vi "fgv_2470-config.vi"(7 "cmd":T2, 11 "2470-config":T1={"Source Mode"=enum."Voltage", "Source Limit Level"=0.01, "Source Level"=0.0, "Output_2470"=FALSE}) -> (3 "2470-config 2":T1)   [LabVIEW 2019]
uses:
  _ctrl/rw.ctl
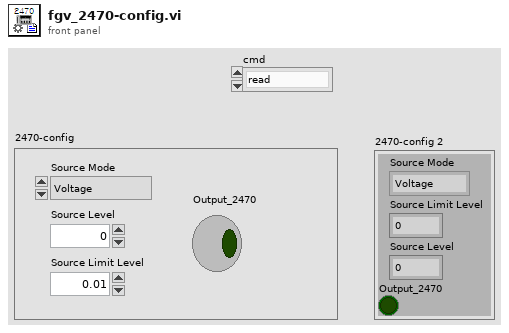
[diagram p1: front panel]
types:
  T1 = cluster{"Source Mode":enum16{"Voltage", "Current"}, "Source Limit Level":dbl, "Source Level":dbl, "Output_2470":bool}
  T2 = typedef "rw.ctl" = enum16{"read", "write"}
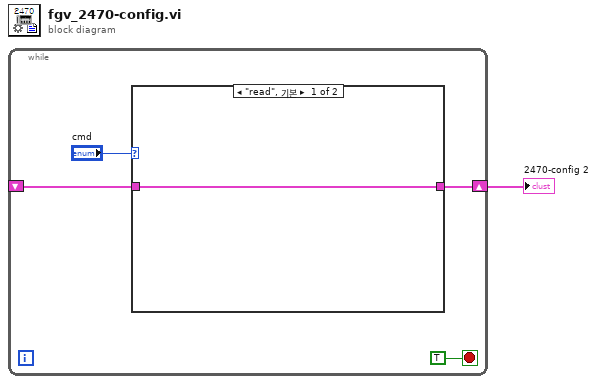
[diagram p0: block diagram]
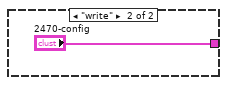
[diagram p2: hidden frame]
diagram:
  n1 = while {
    shift-right: [w3] -> w1
    shift-left: _ -> [w2]
    stop <- TRUE stop-if-true
    n2 = case shown="\"read\", 기본" "cmd" {
      tunnel: [w6 "2470-config"] -> w3
      tunnel: w2 -> [w6 _]
      frame "read", Default {
      }
      frame "write" {
      }
    }
  }
  "2470-config 2" <- w1
